vi "readDefaultILCOutput.vi"(8 "error in (no error)":errorcluster, 11 "Bootloader in":refnum<class "Bootloader.lvclass">) -> (0 "error out":errorcluster, 2 "ILC Outputs":T1 {"Step & Direction" min=-32767}, 3 "Bootloader out":refnum<class "Bootloader.lvclass">)   [LabVIEW 2015, in "Bootloader.lvclass"]
uses:
  Bootloader.lvclass
  <userlib>/Common/ILC/Typedefs/Outputs.ctl
  ConfigurationTestParameters/ConfigurationTestParameters.lvclass
  <userlib>/Common/ILC/Typedefs/ILCTypedefs.lvlib
panel:
  # "DAC"
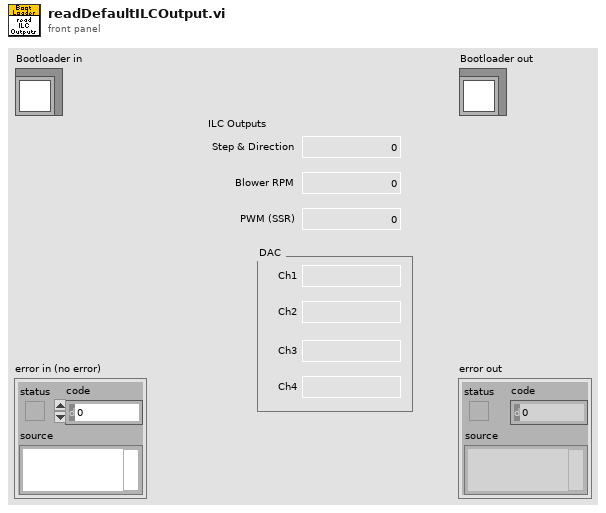
[diagram p1: front panel]
types:
  T1 = typedef "ILCCommon.lvlib/ILCTypedefs.lvlib/Outputs.ctl" = cluster{"Step & Direction":i16, "Blower RPM":u8, "PWM (SSR)":u8, "Ch1":u16, "Ch2":u16, "Ch3":u16, "Ch4":u16}
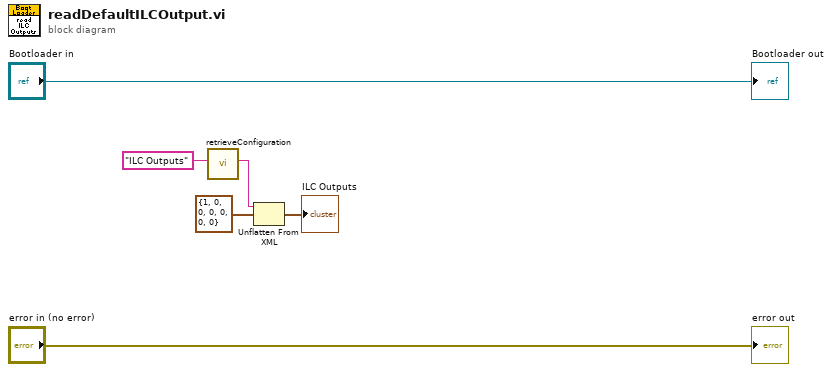
[diagram p0: block diagram]
diagram:
  n1 = call "retrieveConfiguration.vi"("configName"="ILC Outputs") -> ("xmlConfig"=w3:string)  [unwired: 8 in, 2 out]
  n2 = Unflatten From XML(xml string=w3, type=T1 {"Step & Direction"=1, "Blower RPM"=0, "PWM (SSR)"=0, "Ch1"=0, "Ch2"=0, "Ch3"=0, "Ch4"=0} ("ILC Outputs")) -> (value=→"ILC Outputs":T1)  [unwired: 1 in, 1 out]
  "error out" <- "error in (no error)"
  "Bootloader out" <- "Bootloader in"
